vi "Save Config File.vi"(8 "error in (no error)":errorcluster, 11 "Cluster":T1) -> (0 "error out":errorcluster)   [LabVIEW 2017]
uses:
  Controls/Testscreen_Input cluster.ctl
  <vilib>/addons/database/Connection.llb/Conn ObjectReference.ctl
  <vilib>/Utility/config.llb/Write Key (String).vi
  <vilib>/Utility/config.llb/NI_LVConfig.lvlib
  <vilib>/addons/database/NI_Database_API.lvlib
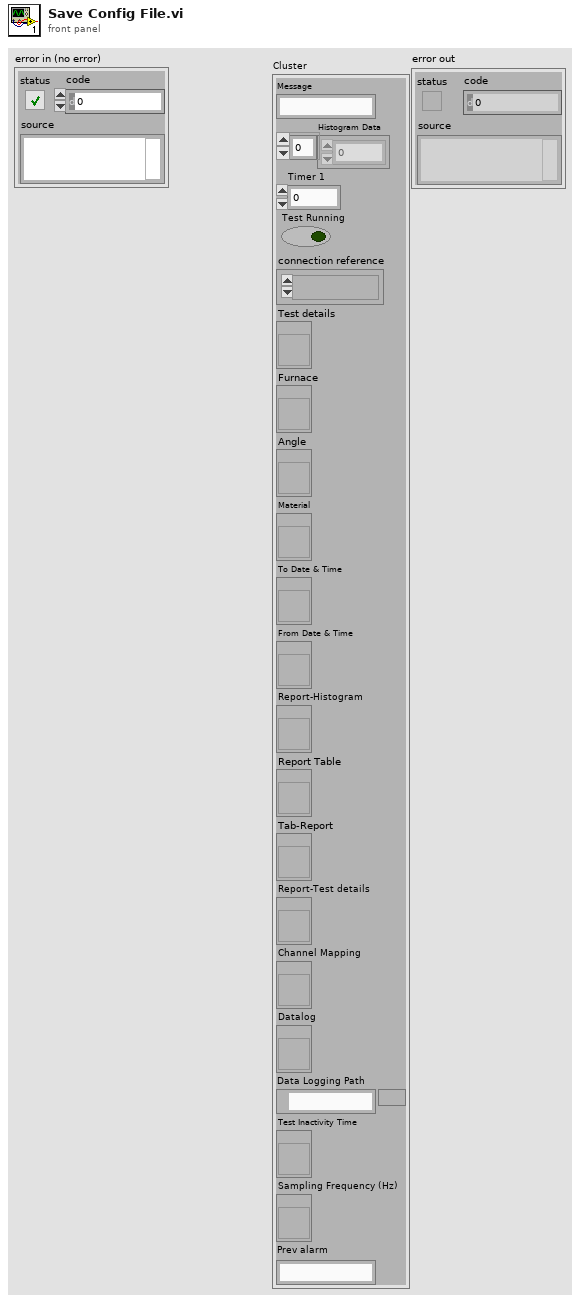
[diagram p1: front panel]
types:
  T1 = typedef "Testscreen_Input cluster.ctl" = cluster{"Message":string, "Histogram Data":i32[], "Timer 1":u32, "Test Running":bool, "connection reference":T2, "Test details":refnum<vi>, "Furnace":refnum<vi>, "Angle":refnum<vi>, "Material":refnum<vi>, "To Date & Time":refnum<vi>, "From Date & Time":refnum<vi>, "Report-Histogram":refnum<vi>, "Report Table":refnum<vi>, "Tab-Report":refnum<vi>, "Report-Test details":refnum<vi>, "Channel Mapping":refnum<vi>, "Datalog":refnum<vi>, "Data Logging Path":path, "Test Inactivity Time":refnum<vi>, "Sampling Frequency (Hz)":refnum<vi>, "Prev alarm":string}
  T2 = typedef "NI_Database_API.lvlib/Conn ObjectReference.ctl" = refnum<k1>
  T3 = cluster{"ID":string, "Test Name":string, "Flowrate":string, "Furnace":string, "Material":string, "Angle":string, "Tested By":string}
  T4 = typedef "NI_LVConfig.lvlib/Config Data RefNum.ctl" = refnum<k1>
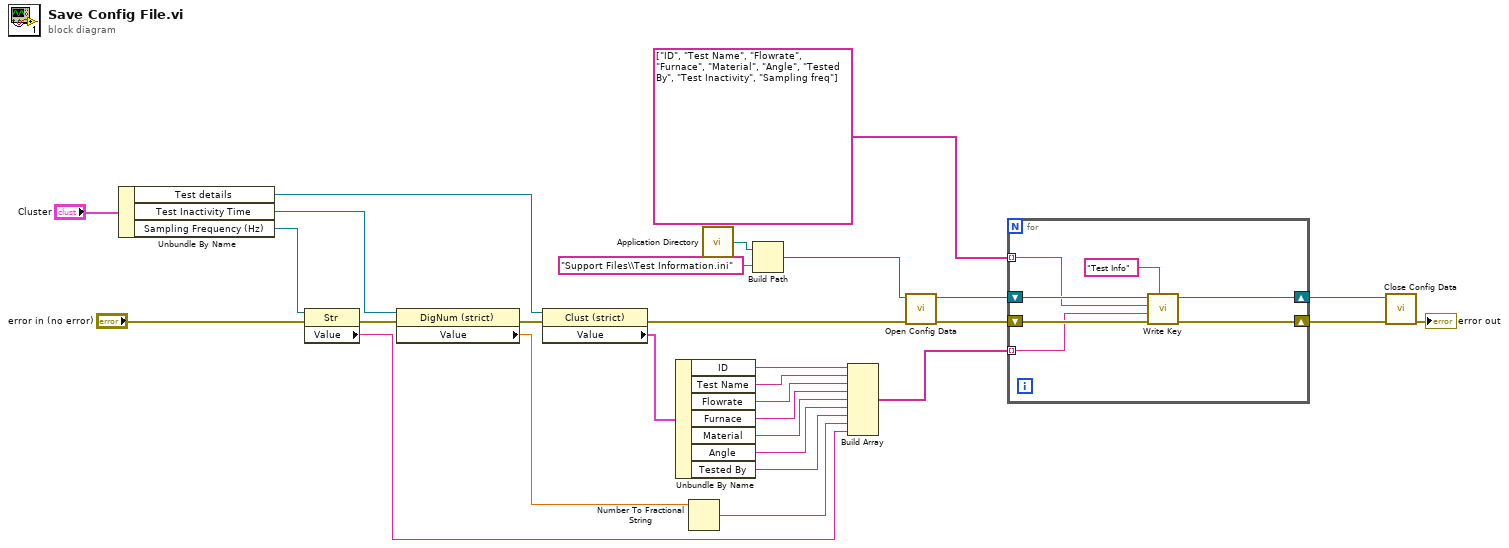
[diagram p0: block diagram]
diagram:
  n1 = Unbundle By Name("Cluster") -> ("Test details"=w14:refnum<vi>, "Test Inactivity Time"=w13:refnum<vi>, "Sampling Frequency (Hz)"=w12:refnum<vi>)
  n2 = property class="Str"(reference=w12, error in="error in (no error)") -> (error out=w11:errorcluster, "Value"=w6:string)  [unwired: 1 out]
  n3 = property class="DigNum (strict)"(reference=w13, error in=w11) -> (error out=w9:errorcluster, "Value"=w8:dbl)  [unwired: 1 out]
  n4 = property class="Clust (strict)"(reference=w14, error in=w9) -> (error out=w16:errorcluster, "Value"=w24:T3)  [unwired: 1 out]
  n5 = Unbundle By Name(w24) -> ("ID"=w17:string, "Test Name"=w18:string, "Flowrate"=w19:string, "Furnace"=w20:string, "Material"=w21:string, "Angle"=w22:string, "Tested By"=w23:string)
  n6 = Number To Fractional String(number=w8) -> (F-format string=w7:string)  [unwired: 3 in]
  n7 = call <vilib>:"Application Directory.vi"() -> ("Application Directory"=w4:path)
  n8 = Build Path(base path=w4, name or relative path="Support Files\\Test Information.ini") -> (appended path=w2:path)
  n9 = Build Array(w17, w18, w19, w20, w21, w22, w23, w7, w6) -> (w5:string[])
  n10 = call <vilib>:"Open Config Data.vi"("error in (no error)"=w16, "configuration file path"=w2) -> ("error out"=w28:errorcluster, "refnum"=w29:T4)  [unwired: 7 in, 1 out]
  n11 = for {
    shift-right: [w33] -> w26
    shift-left: w29 -> [w36]
    shift-right: [w34] -> w27
    shift-left: w28 -> [w35]
    tunnel: string[] ["ID", "Test Name", "Flowrate", "Furnace", "Material", "Angle", "Tested By", "Test Inactivity", "Sampling freq"] ("key") -> [w32] mode=indexing
    tunnel: w5 -> [w31] mode=indexing
    n12 = call-poly <vilib>:"Write Key.vi"("section"="Test Info", "error in (no error)"=w35, "value"=w31, "key"=w32, "refnum"=w36) -> ("error out"=w34:errorcluster, "refnum out"=w33:T4)  [unwired: 4 in, 1 out]
  }
  n13 = call <vilib>:"Close Config Data.vi"("error in (no error)"=w27, "refnum"=w26) -> ("error out"=→"error out":errorcluster)  [unwired: 8 in, 1 out]
